vi "Square Colors.vi"(11 "Map in":refnum<class "Map.lvclass">) -> (2 "Square Colors":u32[][](array[numeric]), 3 "Map out":refnum<class "Map.lvclass">)   [LabVIEW 2020, in "SquareBattle.lvlib" / "Map.lvclass"]
uses:
  Map.lvclass
  Map.lvclass/Map.ctl
  Square/Square.lvclass
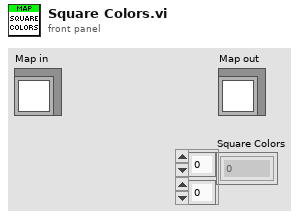
[diagram p1: front panel]
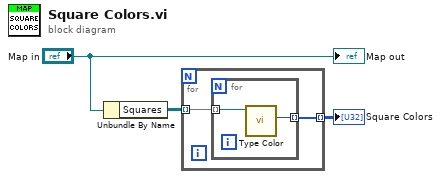
[diagram p0: block diagram]
diagram:
  n1 = Unbundle By Name("Map in") -> ("Squares"=w2:refnum<class "Square.lvclass">[][])
  n2 = for {
    tunnel: w2 -> [w5] mode=indexing
    tunnel: [w4] -> w1 mode=indexing
    n3 = for {
      tunnel: w5 -> [w7] mode=indexing
      tunnel: [w6] -> w4 mode=indexing
      n4 = call-dynamic "Type Color.vi"("Square"=w7) -> ("Type Color"=w6:u32)  [unwired: 10 in]
    }
  }
  "Square Colors" <- w1
  "Map out" <- "Map in"
